vi "ADIS16448 Scale Data_Alt.vi"(8 "error in (no error)":errorcluster, 10 "New Data In":u8[](array[numeric])) -> (0 "error out":errorcluster, 1 "Data Good?":bool, 2 "Data Out":dbl[](array[numeric]))   [LabVIEW 2019]
panel:
  out "Calculated CRC-16":u16
  out "Received CRC-16":u16
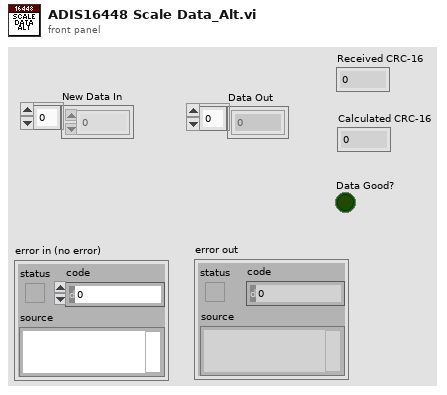
[diagram p1: front panel]
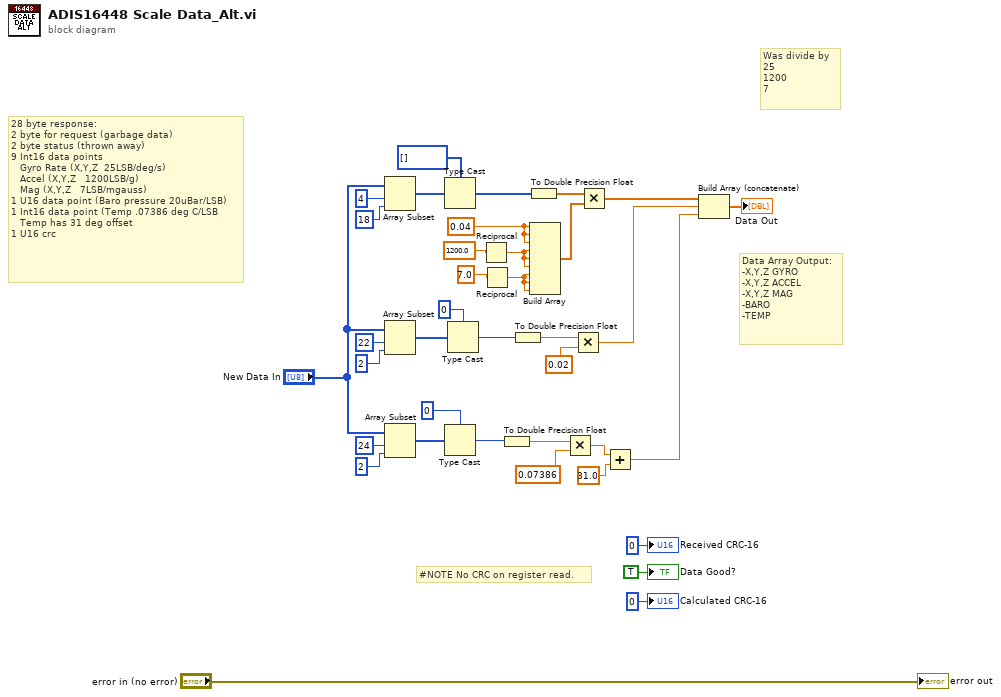
[diagram p0: block diagram]
diagram:
  w1 = 0.04 ("element")
  # "Was divide by \n25\n1200\n7"
  # "#NOTE No CRC on register read."
  # "Data Array Output:\n-X,Y,Z GYRO\n-X,Y,Z ACCEL\n-X,Y,Z MAG\n-BARO\n-TEMP"
  # "28 byte response:\n2 byte for request (garbage data)\n2 byte status (thrown away)\n9 Int16 data points\n   Gyro Rate (X,Y,Z  25LSB/deg/s)\n   Accel (X,Y,Z   1200LSB/g)\n   Mag (X,Y,Z   7LSB/mgauss)\n1 U16 data point (Baro pressure 20uBar/LSB)\n1 Int16 data point (Temp .07386 deg C/LSB\n   Temp has 31 deg offset\n1 U16 crc"
  n1 = Array Subset(array="New Data In", index=4, length=18) -> (w20:u8[])
  n2 = Array Subset(array="New Data In", index=22, length=2) -> (w24:u8[])
  n3 = Array Subset(array="New Data In", index=24, length=2) -> (w22:u8[])
  n4 = Type Cast(type=i16[] [], x=w20) -> (*(type *) &x=w7:i16[])
  n5 = Type Cast(type=i16 0, x=w22) -> (*(type *) &x=w11:i16)
  n6 = Type Cast(type=u16 0, x=w24) -> (*(type *) &x=w9:u16)
  n7 = Reciprocal(x=1200.0) -> (1/x=w3:dbl)
  n8 = Reciprocal(x=7.0) -> (1/x=w2:dbl)
  n9 = To Double Precision Float(number=w11) -> (double precision float=w10:dbl)
  n10 = To Double Precision Float(number=w9) -> (double precision float=w8:dbl)
  n11 = To Double Precision Float(number=w7) -> (double precision float=w6:dbl[])
  n12 = Build Array(w1, w1, w1, w3, w3, w3, w2, w2, w2) -> (w37:dbl[])
  n13 = Multiply(x=w10, y=0.07386 ("element")) -> (x*y=w34:dbl)
  n14 = Multiply(x=w8, y=0.02) -> (x*y=w31:dbl)
  n15 = Multiply(x=w6, y=w37) -> (x*y=w17:dbl[])
  n16 = Add(x=w34, y=31.0) -> (x+y=w32:dbl)
  n17 = Build Array (concatenate)(w17, w31, w32) -> (→"Data Out":dbl[])
  "Received CRC-16" <- u16 0 ("Received CRC-16")
  "Calculated CRC-16" <- u16 0 ("Calculated CRC-16")
  "Data Good?" <- TRUE ("Data Good?")
  "error out" <- "error in (no error)"
